vi "数据流写入.vi"() -> ()   [LabVIEW 2016, in "斯坦道多参数.lvlib"]
panel:
  out "读取方url":string
  in  "停止":bool
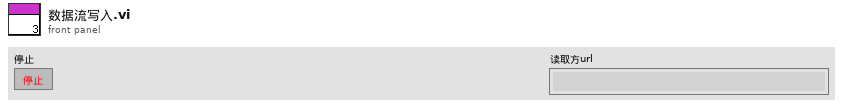
[diagram p1: front panel]
types:
  T1 = typedef "斯坦道多参数.lvlib/数据流类型.ctl" = cluster{"cmd":enum16{"水样测试", "标样核查", "校准状态同步", "停止"}, "data":variant}
  T2 = cluster{"ph":bool, "DO":bool, "Cond":bool, "Turb":bool, "叶绿素a":bool, "藻密度":bool, "ORP":bool, "COD":bool, "DO2":bool, "氯化物":bool, "氨氮":bool, "水中油":bool, "悬浮物":bool, "余氯":bool}
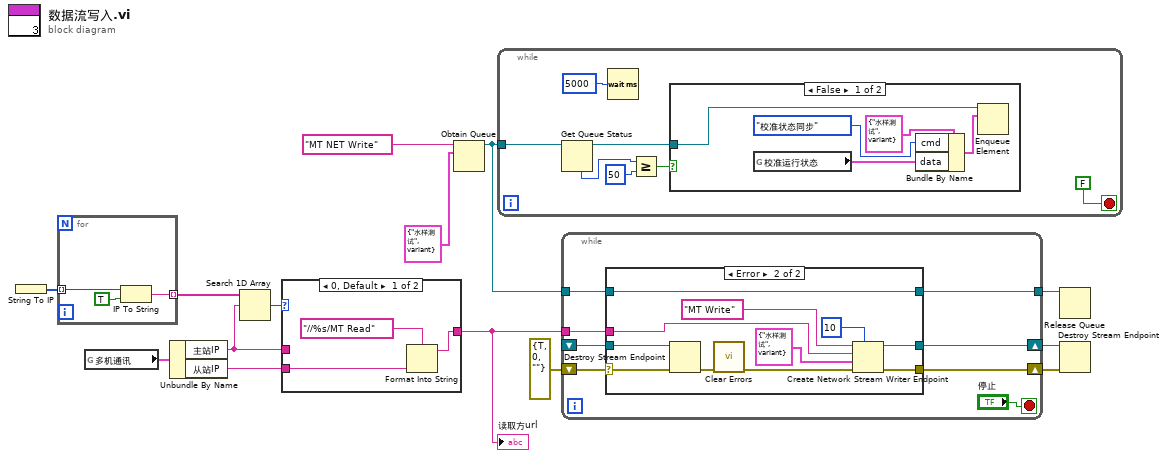
[diagram p0: block diagram]
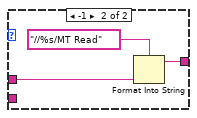
[diagram p2: hidden frame]
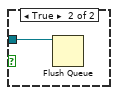
[diagram p3: hidden frame]
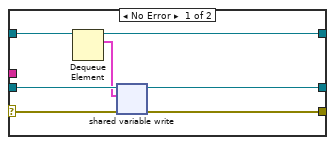
[diagram p4: hidden frame]
diagram:
  n1 = String To IP() -> (0:w3:u32[])  [unwired: 1 in]
  n2 = for {
    tunnel: w3 -> [w17] mode=indexing
    tunnel: [w15] -> w2 mode=indexing
    n3 = IP To String(1:TRUE ("句点符号？(F)"), 2:w17) -> (0:w15:string)
  }
  n4 = global read "断电保存变量.vi" "多机通讯"() -> (w6:cluster{"开启":bool, "主站IP":string, "从站IP":string})
  n5 = Unbundle By Name(w6) -> ("主站IP"=w5:string, "从站IP"=w4:string)
  n6 = Search 1D Array(1D array=w2, element=w5) -> (index of element=w1:i32)  [unwired: 1 in]
  n7 = case shown="0, Default" w1 {
    tunnel: [w19 w21] -> w8
    tunnel: w5 -> [_ w22]
    tunnel: w4 -> [w18 _]
    frame 0, Default {
      n8 = Format Into String(format string="//%s/MT Read" ("格式字符串"), w18) -> (resulting string=w19:string)  [unwired: 2 in, 1 out]
    }
    frame -1 {
      n9 = Format Into String(format string="//%s/MT Read" ("格式字符串"), w22) -> (resulting string=w21:string)  [unwired: 2 in, 1 out]
    }
  }
  "读取方url" <- w8
  n10 = Obtain Queue(name (unnamed)="MT NET Write" ("名称（未命名）"), element data type=T1 {"cmd"=enum."水样测试", "data"=variant} ("簇")) -> (queue out=w9:refnum<queue>)  [unwired: 3 in, 2 out]
  n11 = while {
    tunnel: w9 -> [w30]
    stop <- FALSE stop-if-true
    n12 = Get Queue Status(queue=w30) -> (queue out=w26:refnum<queue>, # elements in queue=w29:i32)  [unwired: 2 in, 6 out]
    n13 = Wait (ms)(milliseconds to wait=u32 5000 ("等待时间（毫秒）")) -> ()  [unwired: 1 out]
    n14 = Greater Or Equal?(x=w29, y=50) -> (x >= y?=w27:bool)
    n15 = case shown="False" w27 {
      tunnel: w26 -> [w35 w36]
      frame False {
        n16 = global read "多参数全局变量.vi" "校准运行状态"() -> (w31:T2)
        n17 = Bundle By Name(cluster=T1 {"cmd"=enum."水样测试", "data"=variant} ("元素"), "cmd"=enum16{"水样测试", "标样核查", "校准状态同步", "停止"}."校准状态同步", "data"=w31) -> (w33:T1)
        n18 = Enqueue Element(queue=w35, element=w33) -> ()  [unwired: 2 in, 3 out]
      }
      frame True {
        n19 = Flush Queue(queue=w36) -> ()  [unwired: 1 in, 3 out]
      }
    }
  }
  n20 = while {
    shift-right: [w44] -> w10
    shift-left: errorcluster {"status"=TRUE, "code"=0, "source"=""} ("error out") -> [w43]
    shift-right: [w42] -> w11
    shift-left: _ -> [w41]
    tunnel: w9 -> [w39]
    tunnel: [w38] -> w12
    tunnel: w8 -> [w37]
    stop <- "停止" stop-if-true
    n21 = case shown="Error" w43 {
      selector: w43 -> [w50 w59]
      tunnel: [w48 w61] -> w44
      tunnel: [w49 w60] -> w42
      tunnel: w41 -> [w51 w58]
      tunnel: w39 -> [w47 w54]
      tunnel: [w45 w54] -> w38
      tunnel: w37 -> [_ w53]
      frame No Error {
        n22 = Dequeue Element(queue=w47) -> (queue out=w45:refnum<queue>, element=w46:T1)  [unwired: 2 in, 2 out]
        n23 = shared-variable-write(w51, w50, w46) -> (w49:refnum<k21>, w48:errorcluster)  [unwired: 1 in, 1 out]
      }
      frame Error {
        n24 = Destroy Stream Endpoint(8:w59, 11:w58) -> (0:w57:errorcluster)
        n25 = call <vilib>:"Clear Errors.vi"("error in (no error)"=w57) -> ("error out"=w56:errorcluster)  [unwired: 5 in, 1 out]
        n26 = Create Network Stream Writer Endpoint(7:10 ("写入方缓冲大小"), 8:w56, 9:T1 {"cmd"=enum."水样测试", "data"=variant} ("簇"), 10:w53, 11:"MT Write" ("写入方名称")) -> (0:w61:errorcluster, 3:w60:refnum<k21>)  [unwired: 2 in]
      }
    }
  }
  n27 = Release Queue(queue=w12) -> ()  [unwired: 2 in, 3 out]
  n28 = Destroy Stream Endpoint(8:w10, 11:w11) -> ()  [unwired: 1 out]
